vi "TimerPrimer.vi"() -> ()   [LabVIEW 2014]
uses:
  Control Timer.ctl
panel:
  in  "stop":bool
  out "Elapsed Time":dbl
  out "Status":cluster{"Running":bool, "Done":bool}
  in  "OK Button":bool
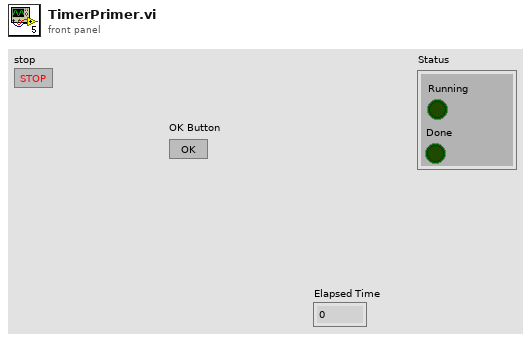
[diagram p1: front panel]
types:
  T1 = typedef "Control Timer.ctl" = enum16{"Timecheck", "Reset"}
  T2 = typedef "Control Timer.ctl" = enum16{"Timecheck", "Reset", "Pause"}
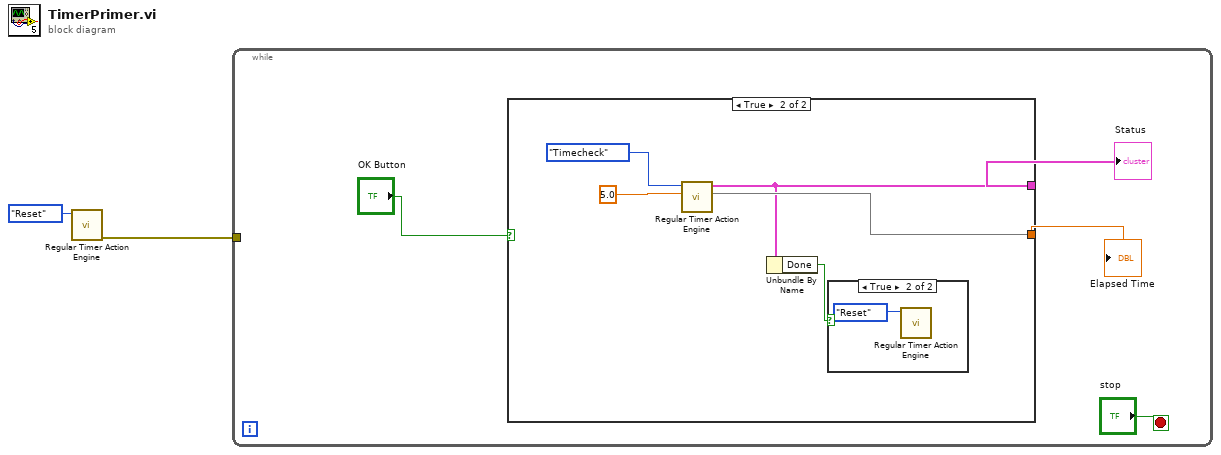
[diagram p0: block diagram]
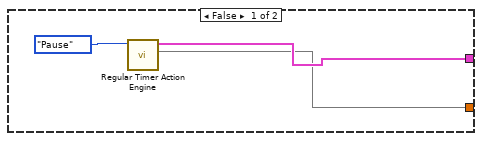
[diagram p2: hidden frame]
diagram:
  n1 = call "Regular Timer Action Engine.vi"("Enum"=Control_Timer."Reset") -> ("error out"=w1:errorcluster)  [unwired: 8 in, 1 out]
  n2 = while {
    tunnel: w1 -> [_]
    stop <- "stop" stop-if-true
    n3 = case shown="True" "OK Button" {
      tunnel: [w8 w11] -> w5
      tunnel: [w7 w13] -> w4
      frame False {
        n4 = call "Regular Timer Action Engine.vi"("Enum"=Control_Timer."Pause") -> ("Status"=w8:cluster{"Running":bool, "Done":bool}, 8:w7)  [unwired: 7 in, 1 out]
      }
      frame True {
        n5 = call "Regular Timer Action Engine.vi"("Enum"=Control_Timer."Timecheck", "Time Target"=5.0) -> ("Status"=w11:cluster{"Running":bool, "Done":bool}, 8:w13)  [unwired: 6 in, 1 out]
        n6 = Unbundle By Name(w11) -> ("Done"=w10:bool)
        n7 = case shown="True" w10 {
          frame False {
          }
          frame True {
            n8 = call "Regular Timer Action Engine.vi"("Enum"=Control_Timer."Reset") -> ()  [unwired: 8 in, 2 out]
          }
        }
      }
    }
    "Status" <- w5
    "Elapsed Time" <- w4
  }
